vi "UpdateListBoxAfterKeyEvent.vi"(7 "DiscardEvent?":bool, 8 "error in (no error)":errorcluster, 10 "VKey":T2, 11 "control refs":T1) -> (0 "error out":errorcluster)   [LabVIEW 2017]
uses:
  <vilib>/event_ctls.llb/eventvkey.ctl
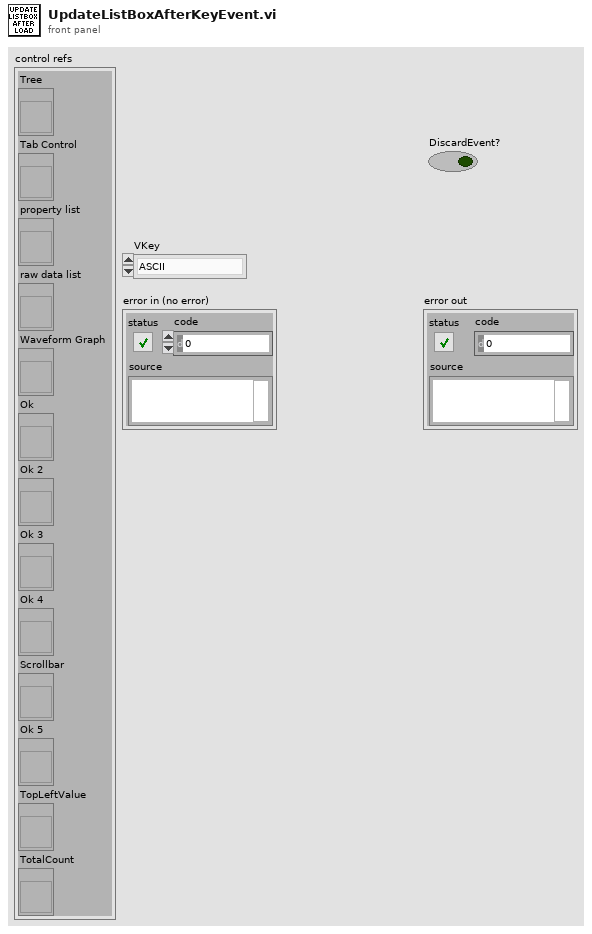
[diagram p1: front panel]
types:
  T1 = cluster{"Tree":refnum<vi>, "Tab Control":refnum<vi>, "property list":refnum<vi>, "raw data list":refnum<vi>, "Waveform Graph":refnum<vi>, "Ok":refnum<vi>, "Ok 2":refnum<vi>, "Ok 3":refnum<vi>, "Ok 4":refnum<vi>, "Scrollbar":refnum<vi>, "Ok 5":refnum<vi>, "TopLeftValue":refnum<vi>, "TotalCount":refnum<vi>}
  T2 = typedef "eventvkey.ctl" = enum16{"ASCII", "Enter", "Return", "Shift", "Ctrl", "Alt", "Cmd", "Opt", "Caps", "NumLock", "Clear", "Break", "Up", "Down", "Left", "Right", "Insert", "Delete", "Home", "End", "PageUp", "PageDown", "Escape", "Help", "Pause", "ScrollLock", "F1", "F2", "F3", "F4", "F5", "F6", "F7", "F8", "F9", "F10", "F11", "F12", "F13", "F14", "F15", "F16", "F17", "F18", "F19", "F20", "F21", "F22", "F23", "F24", "Play", "VolumeUp", "VolumeDown", "Mute", "Two Byte Char"}
  T3 = typedef "LVRowAndColumnUnsignedTypeDef.ctl" = cluster{"Row":u32, "Column":u32}
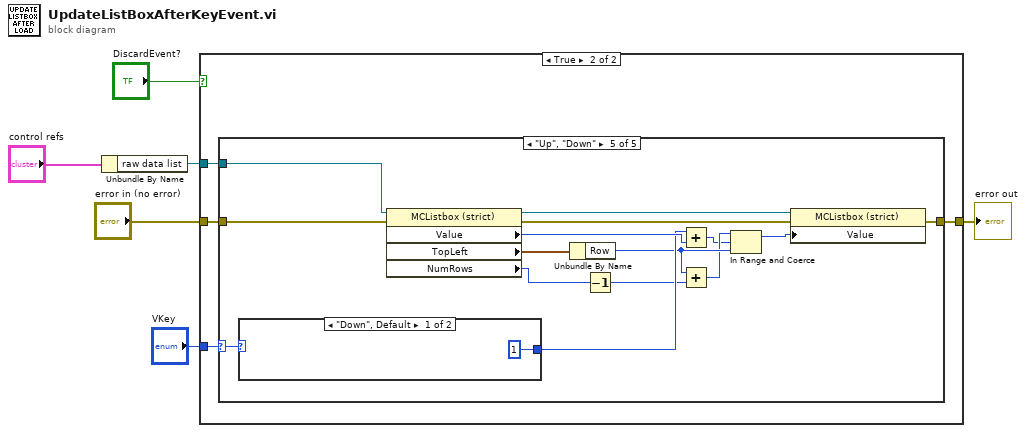
[diagram p0: block diagram]
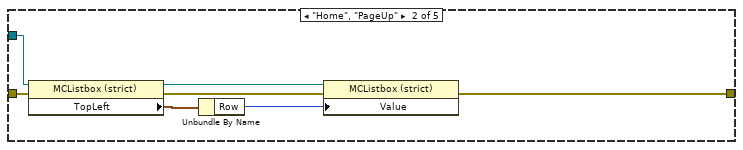
[diagram p4: hidden frame]
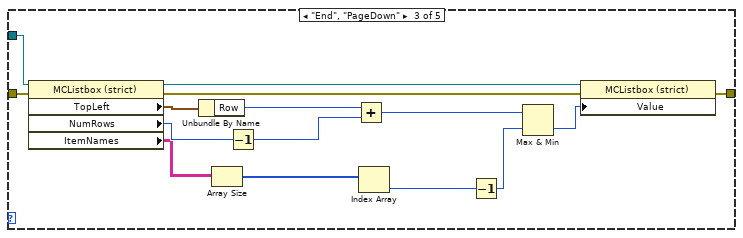
[diagram p5: hidden frame]
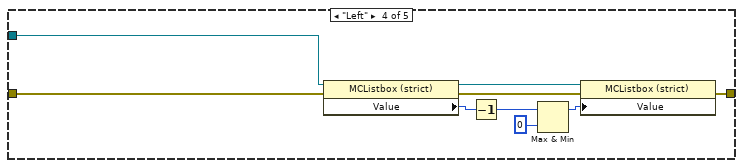
[diagram p6: hidden frame]
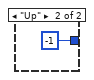
[diagram p7: hidden frame]
diagram:
  n1 = Unbundle By Name("control refs") -> ("raw data list"=w2:refnum<vi>)
  n2 = case shown="True" "DiscardEvent?" {
    tunnel: "error in (no error)" -> [w7 w11]
    tunnel: [w7 w10] -> w4
    tunnel: "VKey" -> [_ w9]
    tunnel: w2 -> [_ w8]
    frame False {
    }
    frame True {
      n3 = case shown="\"Up\", \"Down\"" w9 {
        selector: w9 -> [_ _ _ _ w55]
        tunnel: w11 -> [w12 w18 w24 w42 w57]
        tunnel: [w12 w19 w34 w43 w58] -> w10
        tunnel: w8 -> [_ w14 w31 w40 w56]
        frame Default {
        }
        frame "Home", "PageUp" {
          n4 = property on="Property Node" class="MCListbox (strict)"(reference=w14, error in=w18) -> (reference out=w13:refnum<vi>, error out=w16:errorcluster, "TopLeft"=w17:T3)
          n5 = Unbundle By Name(w17) -> ("Row"=w15:u32)
          n6 = property on="Property Node" class="MCListbox (strict)"(reference=w13, error in=w16, "Value"=w15) -> (error out=w19:errorcluster)  [unwired: 1 out]
        }
        frame "End", "PageDown" {
          n7 = property on="Property Node" class="MCListbox (strict)"(reference=w31, error in=w24) -> (reference out=w30:refnum<vi>, error out=w32:errorcluster, "TopLeft"=w33:T3, "NumRows"=w28:u32, "ItemNames"=w23:string[][])
          n8 = Unbundle By Name(w33) -> ("Row"=w29:u32)
          n9 = Array Size(array=w23) -> (size(s)=w22:i32[])
          n10 = Decrement(x=w28) -> (x-1=w27:u32)
          n11 = Add(x=w29, y=w27) -> (x+y=w26:u32)
          n12 = Index Array(array=w22) -> (element=w21:i32)  [unwired: 1 in]
          n13 = Decrement(x=w21) -> (x-1=w20:i32)
          n14 = Max & Min(x=w26, y=w20) -> (min(x,y)=w25:u32)  [unwired: 1 out]
          n15 = property on="Property Node" class="MCListbox (strict)"(reference=w30, error in=w32, "Value"=w25) -> (error out=w34:errorcluster)  [unwired: 1 out]
        }
        frame "Left" {
          n16 = property on="Property Node" class="MCListbox (strict)"(reference=w40, error in=w42) -> (reference out=w39:refnum<vi>, error out=w41:errorcluster, "Value"=w38:i32)
          n17 = Decrement(x=w38) -> (x-1=w37:i32)
          n18 = Max & Min(x=w37, y=0) -> (max(x,y)=w35:i32)  [unwired: 1 out]
          n19 = property on="Property Node" class="MCListbox (strict)"(reference=w39, error in=w41, "Value"=w35) -> (error out=w43:errorcluster)  [unwired: 1 out]
        }
        frame "Up", "Down" {
          n20 = case shown="\"Down\", Default" w55 {
            tunnel: [i64 1 i64 -1] -> w53
            frame "Down", Default {
            }
            frame "Up" {
            }
          }
          n21 = property on="Property Node" class="MCListbox (strict)"(reference=w56, error in=w57) -> (reference out=w51:refnum<vi>, error out=w50:errorcluster, "Value"=w54:i32, "TopLeft"=w52:T3, "NumRows"=w45:u32)
          n22 = Unbundle By Name(w52) -> ("Row"=w49:u32)
          n23 = Decrement(x=w45) -> (x-1=w44:u32)
          n24 = Add(x=w53, y=w54) -> (x+y=w47:i64)
          n25 = Add(x=w49, y=w44) -> (x+y=w48:u32)
          n26 = In Range and Coerce(upper limit=w48, x=w47, lower limit=w49) -> (coerced(x)=w46:i64)  [unwired: 1 out]
          n27 = property on="Property Node" class="MCListbox (strict)"(reference=w51, error in=w50, "Value"=w46) -> (error out=w58:errorcluster)  [unwired: 1 out]
        }
      }
    }
  }
  "error out" <- w4
